vi "OpenDataLogFileForWriting.vi"(0 "Filename":string) -> (1 "Data Log File Refnum":refnum<k1>, 2 "error out":errorcluster)   [LabVIEW 2011]
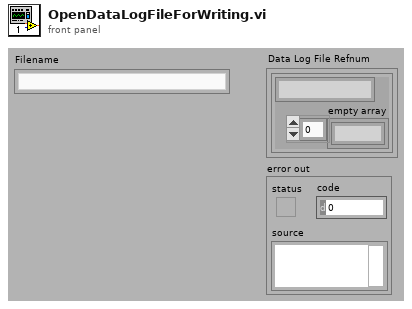
[diagram p1: front panel]
types:
  T1 = enum16{"open", "replace", "create", "open or create", "replace or create", "replace or create with confirmation"}
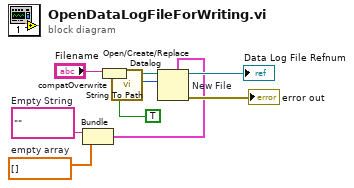
[diagram p0: block diagram]
diagram:
  w9 = ""  # Empty String
  w8 = sgl[] []  # empty array
  n1 = Bundle(w9, "empty array"=w8) -> (w4:cluster{string, "empty array":sgl[]})  [unwired: 1 out]
  n2 = String To Path(string="Filename") -> (path=w2:path)
  n3 = call <vilib>:"compatOverwrite.vi"("overwrite (F)"=TRUE) -> ("overwrite?"=w1:T1)
  n4 = Open/Create/Replace Datalog "New File"(5:w4, 10:w1, 11:w2) -> (0:→"error out":errorcluster, 3:→"Data Log File Refnum":refnum<k1>)  [unwired: 1 in, 3 out]
